vi "Get All Tags.vi"(7 "Filter (none)":string, 8 "error in (no error)":errorcluster) -> (0 "error out":errorcluster, 1 "Tag Refs":refnum<data-value>[](array[refnum]), 2 "Tag Names":string[](array[string]))   [LabVIEW 2018, in "Tag Engine.lvlib" / "Tag Core.lvclass"]
doc: "Return a list of all CVT item names and references.\n\nOptionally specify a filter. Only matched item names will be returned. Standard \"Match Pattern\" syntax applies. Match is not case sensitive."
uses:
  Tag Core.lvclass
  Tag/Tag.lvclass
  Tag Core.lvclass/Tag Core.ctl
  Tag/Tag.lvclass/Tag.ctl
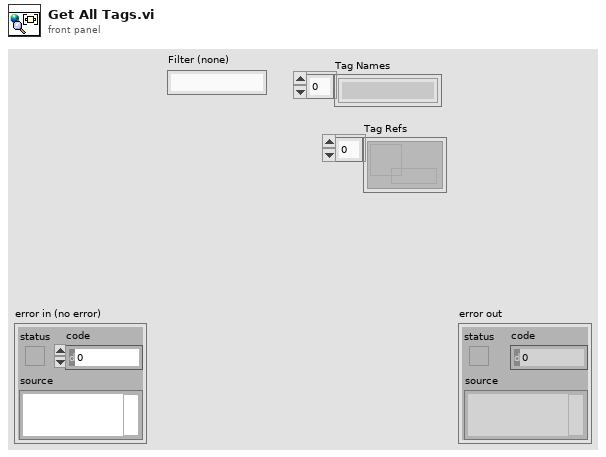
[diagram p1: front panel]
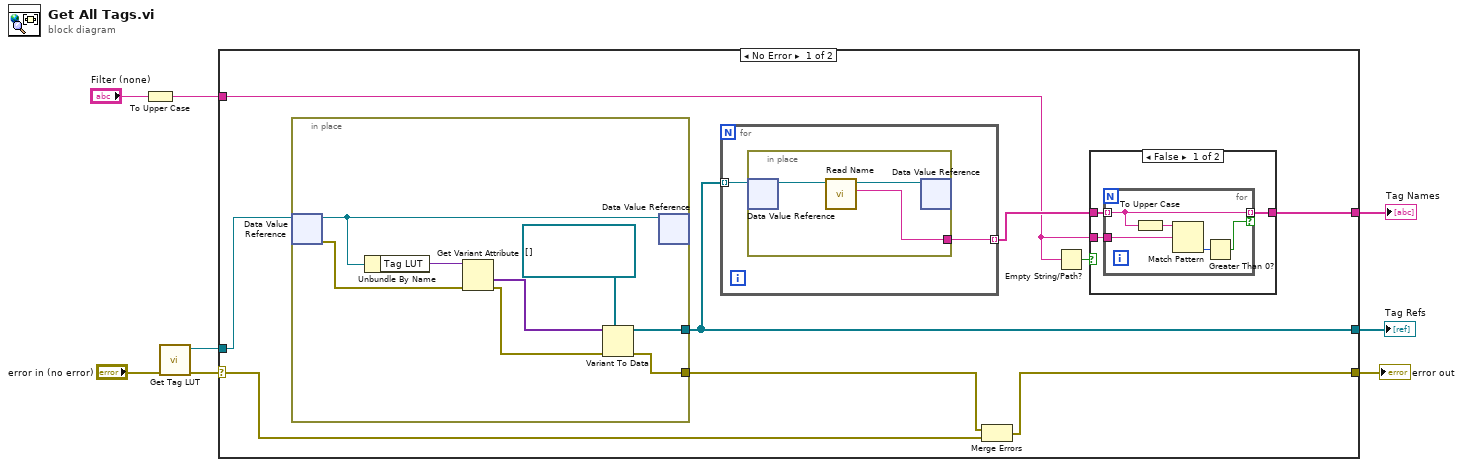
[diagram p0: block diagram]
diagram:
  n1 = To Upper Case(1:"Filter (none)") -> (0:w1:string)
  n2 = call "Get Tag LUT.vi"("error in (no error)"="error in (no error)") -> ("error out"=w6:errorcluster, "Tag LUT Out"=w5:refnum<data-value>)  [unwired: 9 in]
  n3 = case shown="No Error" w6 {
    selector: w6 -> [w16 w40]
    tunnel: [w14 w40] -> w8
    tunnel: w5 -> [w17 _]
    tunnel: [w9 _] -> w3
    tunnel: [w13 _] -> w4
    tunnel: w1 -> [w10 _]
    frame No Error {
      n4 = in-place {
        in-place-border: [w35] -> w13
        in-place-border: [w32] -> w15
        n5 = in-place-dvr #1(w17) -> (w39:refnum<class "Tag Core.lvclass">, w34:errorcluster)
        n6 = Unbundle By Name(w39) -> ("Tag LUT"=w38:variant)
        n7 = Get Variant Attribute(Variant=w38, error in=w34) -> (values=w37:variant[], error out=w33:errorcluster)  [unwired: 2 in, 2 out]
        n8 = Variant To Data(error in=w33, type=refnum<data-value>[] [] ("CVT Item in"), Variant=w37) -> (data=w35:refnum<data-value>[], error out=w32:errorcluster)
        n9 = in-place-dvr #1(w39) -> ()  [unwired: 2 out]
      }
      n10 = for {
        tunnel: w13 -> [w28] mode=indexing
        tunnel: [w27] -> w11 mode=indexing
        n11 = in-place {
          in-place-border: [w29] -> w27
          n12 = in-place-dvr #2(w28) -> (w31:refnum<class "Tag.lvclass">)  [unwired: 1 out]
          n13 = call "Read Name.vi"("Tag in"=w31) -> ("Name"=w29:string, "Tag out"=w30:refnum<class "Tag.lvclass">)  [unwired: 8 in, 1 out]
          n14 = in-place-dvr #2(w30) -> ()  [unwired: 2 out]
        }
      }
      n15 = Merge Errors(w15, w16) -> (w14:errorcluster)
      n16 = Empty String/Path?(string/path=w10) -> (empty?=w12:bool)
      n17 = case shown="False" w12 {
        tunnel: w11 -> [w20 w26]
        tunnel: [w19 w26] -> w9
        tunnel: w10 -> [w18 _]
        frame False {
          n18 = for {
            tunnel: w18 -> [w25]
            tunnel: w20 -> [w22] mode=indexing
            tunnel: [w22] -> w19 mode=indexing if=w23
            n19 = To Upper Case(1:w22) -> (0:w21:string)
            n20 = Match Pattern(string=w21, regular expression=w25) -> (offset past match=w24:i32)  [unwired: 1 in, 3 out]
            n21 = Greater Than 0?(x=w24) -> (x > 0?=w23:bool)
          }
        }
        frame True {
        }
      }
    }
    frame Error {
    }
  }
  "error out" <- w8
  "Tag Refs" <- w4
  "Tag Names" <- w3
